vi "Read Status.vi"(8 "error in (no error)":errorcluster, 11 "Comdel in":refnum<class "PL Comdel CX.lvclass">) -> (0 "error out":errorcluster, 2 "status":T1, 3 "Comdel out":refnum<class "PL Comdel CX.lvclass">)   [LabVIEW 2015, in "PL Comdel CX.lvclass"]
doc: "Reads device <b>status</b>."
uses:
  PL Comdel CX.lvclass
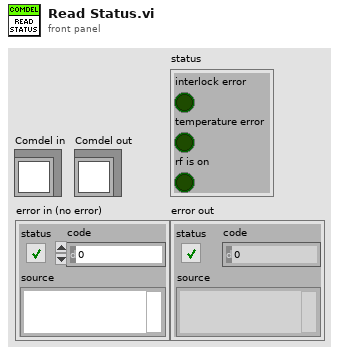
[diagram p1: front panel]
types:
  T1 = cluster{"interlock error":bool, "temperature error":bool, "rf is on":bool}
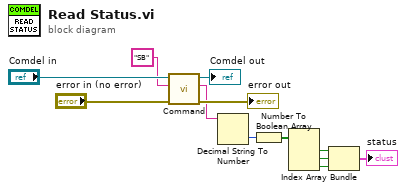
[diagram p0: block diagram]
diagram:
  n1 = call "Command.vi"("error in (no error)"="error in (no error)", "command"="SB", "Comdel in"="Comdel in") -> ("error out"=→"error out":errorcluster, "response data"=w7:string, "Comdel out"=→"Comdel out":refnum<class "PL Comdel CX.lvclass">)  [unwired: 6 in]
  n2 = Decimal String To Number(string=w7) -> (number=w6:i32)  [unwired: 2 in, 1 out]
  n3 = Number To Boolean Array(number=w6) -> (Boolean array=w5:bool[])
  n4 = Index Array(array=w5) -> (element #1=w4:bool, element #2=w2:bool, element #3=w3:bool)  [unwired: 3 in]
  n5 = Bundle(w4, w2, w3) -> (→"status":cluster{bool, bool, bool})  [unwired: 1 in]
